vi "Disconnect.vi"(8 "error in (no error)":errorcluster, 10 "Disconnection list in":string, 11 "SLSC Switch Consumer in":refnum<class "SLSC Switch Consumer.lvclass">) -> (0 "error out":errorcluster, 3 "SLSC Switch Consumer out":refnum<class "SLSC Switch Consumer.lvclass">)   [LabVIEW 2017, in "SLSC Switch Messaging.lvlib" / "SLSC Switch Consumer.lvclass"]
uses:
  SLSC Switch Consumer.lvclass
  SLSC Switch Consumer.lvclass/SLSC Switch Consumer.ctl
  <vilib>/SLSC_Switch/Disconnect Channels (Multiple).vi
  <vilib>/SLSC_Switch/SLSC Switch.lvlib
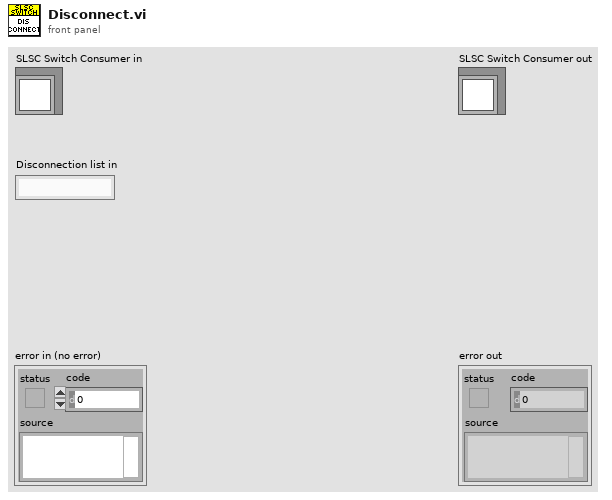
[diagram p1: front panel]
types:
  T1 = typedef "nislscslSession.ctl" = refnum<k20>
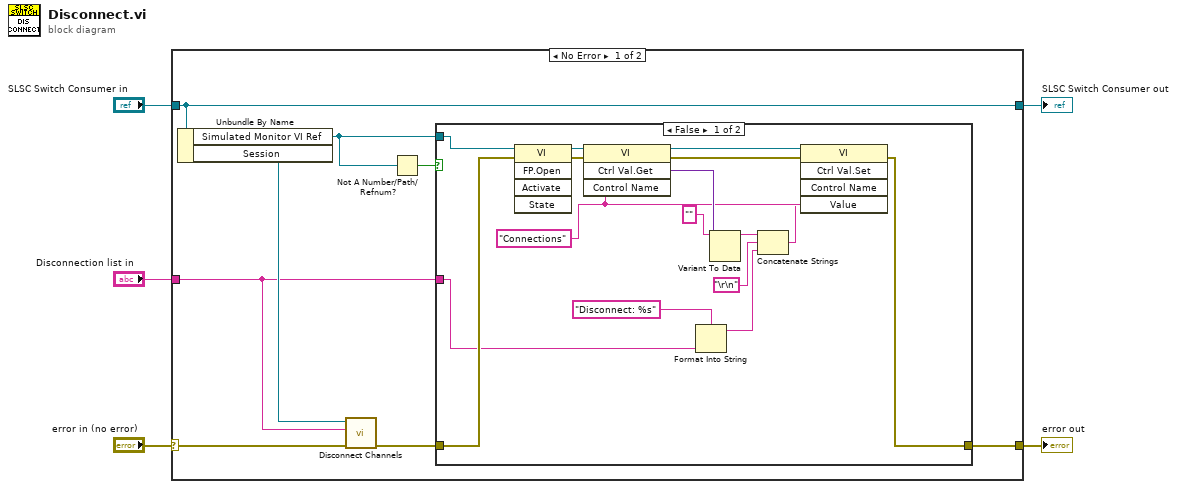
[diagram p0: block diagram]
diagram:
  n1 = case shown="No Error" "error in (no error)" {
    selector: "error in (no error)" -> [w11 w32]
    tunnel: [w6 w32] -> w3
    tunnel: [w13 w31] -> w1
    tunnel: "SLSC Switch Consumer in" -> [w13 w31]
    tunnel: "Disconnection list in" -> [w8 _]
    frame No Error {
      n2 = Unbundle By Name(w13) -> ("Simulated Monitor VI Ref"=w9:refnum<vi>, "Session"=w12:T1)
      n3 = call-poly <vilib>:"Disconnect Channels.vi"("error in (no error)"=w11, "disconnection list"=w8, "session in"=w12) -> ("error out"=w7:errorcluster)  [unwired: 7 in, 1 out]
      n4 = Not A Number/Path/Refnum?(number/path/refnum=w9) -> (NaN/Path/Refnum?=w10:bool)
      n5 = case shown="False" w10 {
        tunnel: w9 -> [w15 _]
        tunnel: w8 -> [w19 _]
        tunnel: w7 -> [w29 w30]
        tunnel: [w26 w30] -> w6
        frame False {
          w21 = "Connections" ("Control Name")
          n6 = invoke class="VI" method="FP.Open"(reference=w15, error in=w29) -> (reference out=w14:refnum<vi>, error out=w28:errorcluster)  [unwired: 3 in, 3 out]
          n7 = invoke class="VI" method="Ctrl Val.Get"(reference=w14, error in=w28, "Control Name"=w21) -> (reference out=w27:refnum<vi>, error out=w16:errorcluster, "Get Control Value Variant"=w25:variant)  [unwired: 1 in, 1 out]
          n8 = Format Into String(format string="Disconnect: %s" ("Control Name"), w19) -> (resulting string=w18:string)  [unwired: 2 in, 1 out]
          n9 = Variant To Data(type="" ("Control Name"), Variant=w25) -> (data=w23:string)  [unwired: 1 in, 1 out]
          n10 = Concatenate Strings(w23, "\r\n", w18) -> (w17:string)
          n11 = invoke class="VI" method="Ctrl Val.Set"(reference=w27, error in=w16, "Control Name"=w21, "Value"=w17) -> (error out=w26:errorcluster)  [unwired: 1 in, 4 out]
        }
        frame True {
        }
      }
    }
    frame Error {
    }
  }
  "error out" <- w3
  "SLSC Switch Consumer out" <- w1
